vi "(SubVI) SaveTxtHeader-time.vi"(10 "Select a Folder":path, 11 "Time Axis (s)":dbl[](array[numeric])) -> ()   [LabVIEW 2014]
uses:
  <vilib>/Utility/file.llb/Write To Spreadsheet File (string).vi
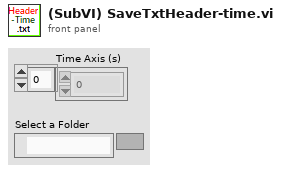
[diagram p1: front panel]
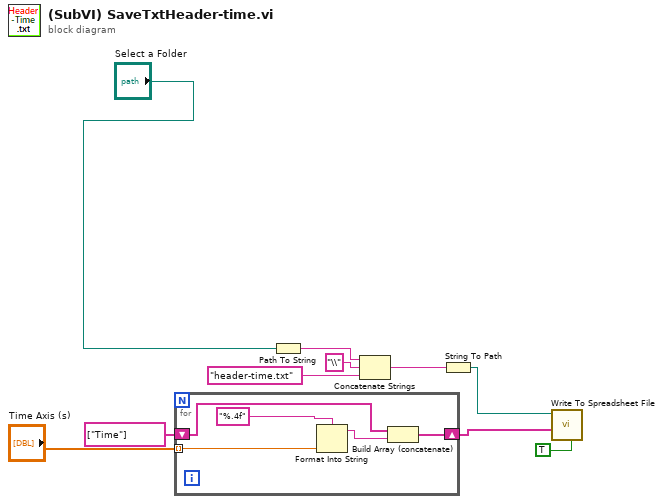
[diagram p0: block diagram]
diagram:
  n1 = for {
    tunnel: "Time Axis (s)" -> [w14] mode=indexing
    shift-right: [w12] -> w3
    shift-left: string[] ["Time"] -> [w11]
    n2 = Format Into String(format string="%.4f" ("initial string"), w14) -> (resulting string=w13:string)  [unwired: 2 in, 1 out]
    n3 = Build Array (concatenate)(w11, w13) -> (w12:string[])
  }
  n4 = Path To String(path="Select a Folder") -> (string=w6:string)
  n5 = Concatenate Strings(w6, "\\" ("string"), "header-time.txt" ("string")) -> (w7:string)
  n6 = String To Path(string=w7) -> (path=w10:path)
  n7 = call-poly <vilib>:"Write To Spreadsheet File.vi"("transpose? (no:F)"=TRUE, "1D data"=w3, "file path (dialog if empty)"=w10) -> ()  [unwired: 5 in, 1 out]
